vi "ACQ Read.vi"(8 "error in (no error)":errorcluster, 11 "VISA resource name In":T1={"Conection Data"="COM4"}) -> (0 "error out":errorcluster, 2 "Value":sgl format="%.2f", 3 "VISA resource name Out":T1={"Conection Data"="COM4"})   [LabVIEW 2014, in "AD4212C Lib.lvlib"]
doc: "Lee los datos del Buffer, detecta errores e inestabilidades de la adquisición. Convierte los datos a formato SGL."
uses:
  AD4212C Lib.lvlib
  Typedef/Connection Data.ctl
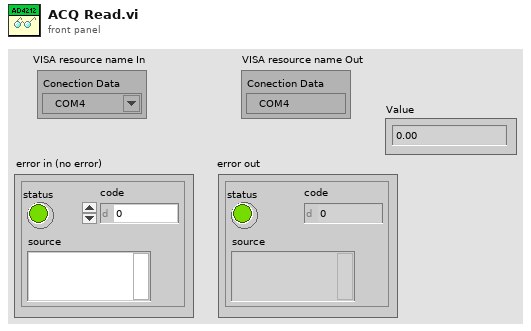
[diagram p1: front panel]
types:
  T1 = typedef "AD4212C Lib.lvlib/Connection Data.ctl" = cluster{"Conection Data":refnum<visa-resource-name>}
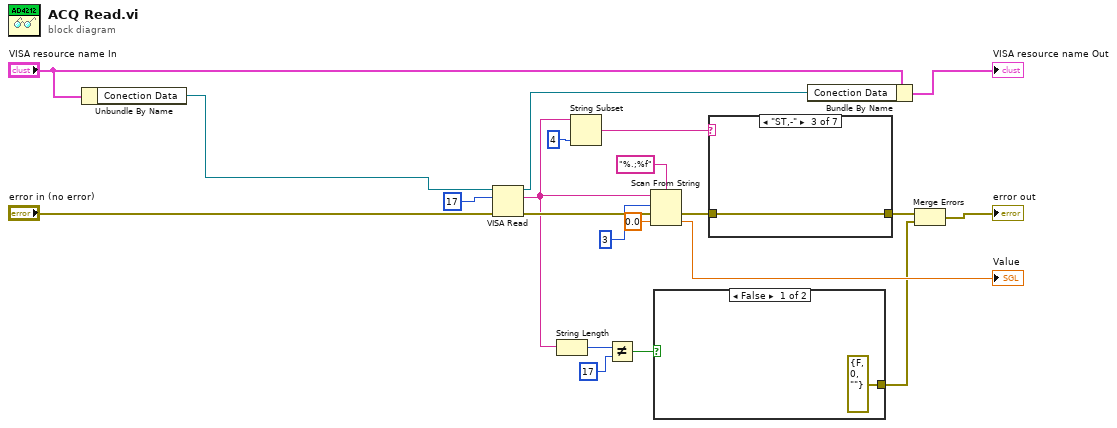
[diagram p0: block diagram]
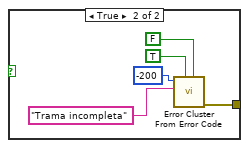
[diagram p2: hidden frame]
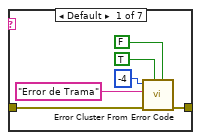
[diagram p3: hidden frame]
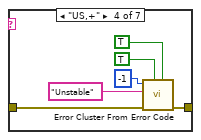
[diagram p5: hidden frame]
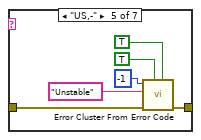
[diagram p6: hidden frame]
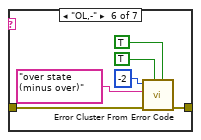
[diagram p7: hidden frame]
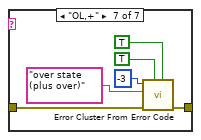
[diagram p8: hidden frame]
diagram:
  n1 = Unbundle By Name("VISA resource name In") -> ("Conection Data"=w2:refnum<visa-resource-name>)
  n2 = VISA Read(VISA resource name=w2, byte count=u32 17 ("バイトカウント（0）"), error in (no error)="error in (no error)") -> (VISA resource name out=w10:refnum<visa-resource-name>, read buffer=w9:string, error out=w16:errorcluster)  [unwired: 1 out]
  n3 = String Length(string=w9) -> (length=w8:i32)
  n4 = String Subset(string=w9, length (rest)=4 ("長さ（残り）")) -> (substring=w14:string)  [unwired: 1 in]
  n5 = Not Equal?(x=w8, y=17) -> (x != y?=w6:bool)
  n6 = Scan From String(format string="%.;%f", input string=w9, initial scan location=u32 3 ("初期スキャン位置"), error in=w16, default 1=sgl 0.0 ("default value 1")) -> (error out=w12:errorcluster, output 1=→"Value":sgl)  [unwired: 2 out]
  n7 = case shown="False" w6 {
    tunnel: [errorcluster {"status"=FALSE, "code"=0, "source"=""} ("error out") w23] -> w5
    frame False {
    }
    frame True {
      n8 = call <vilib>:"Error Cluster From Error Code.vi"("is warning? (False)"=FALSE, "show call chain? (False)"=TRUE ("is warning? (False)"), "error message (\"\")"="Trama incompleta" ("error message (\"\")"), "error code (0)"=-200) -> ("error out"=w23:errorcluster)  [unwired: 5 in]
    }
  }
  n9 = case shown="\"ST,-\"" w14 {
    tunnel: [w33 w34 w35 w40 w46 w53 w58] -> w4
    tunnel: w12 -> [w32 w34 w35 w41 w47 w52 w59]
    frame Default {
      n10 = call <vilib>:"Error Cluster From Error Code.vi"("is warning? (False)"=FALSE, "show call chain? (False)"=TRUE, "error in (no error)"=w32, "error message (\"\")"="Error de Trama" ("error message (\"\")"), "error code (0)"=-4) -> ("error out"=w33:errorcluster)  [unwired: 4 in]
    }
    frame "ST,+" {
    }
    frame "ST,-" {
    }
    frame "US,+" {
      n11 = call <vilib>:"Error Cluster From Error Code.vi"("is warning? (False)"=TRUE, "show call chain? (False)"=TRUE ("is warning? (False)"), "error in (no error)"=w41, "error message (\"\")"="Unstable" ("error message (\"\")"), "error code (0)"=-1) -> ("error out"=w40:errorcluster)  [unwired: 4 in]
    }
    frame "US,-" {
      n12 = call <vilib>:"Error Cluster From Error Code.vi"("is warning? (False)"=TRUE, "show call chain? (False)"=TRUE ("is warning? (False)"), "error in (no error)"=w47, "error message (\"\")"="Unstable" ("error message (\"\")"), "error code (0)"=-1) -> ("error out"=w46:errorcluster)  [unwired: 4 in]
    }
    frame "OL,-" {
      n13 = call <vilib>:"Error Cluster From Error Code.vi"("is warning? (False)"=TRUE, "show call chain? (False)"=TRUE, "error in (no error)"=w52, "error message (\"\")"="over state (minus over)" ("error message (\"\")"), "error code (0)"=-2) -> ("error out"=w53:errorcluster)  [unwired: 4 in]
    }
    frame "OL,+" {
      n14 = call <vilib>:"Error Cluster From Error Code.vi"("is warning? (False)"=TRUE, "show call chain? (False)"=TRUE ("is warning? (False)"), "error in (no error)"=w59, "error message (\"\")"="over state (plus over)" ("error message (\"\")"), "error code (0)"=-3) -> ("error out"=w58:errorcluster)  [unwired: 4 in]
    }
  }
  n15 = Bundle By Name(cluster="VISA resource name In", "Conection Data"=w10) -> (→"VISA resource name Out":T1)
  n16 = Merge Errors(w4, w5) -> (→"error out":errorcluster)
